vi "Write Start Meas.vi"(8 "error in (no error)":errorcluster, 10 "Start Meas":bool, 11 "Control-Client in":refnum<class "Control-Client.lvclass">) -> (0 "error out":errorcluster, 3 "Control-Client out":refnum<class "Control-Client.lvclass">)   [LabVIEW 2015, in "Control-Client.lvclass"]
uses:
  Control-Client.lvclass
  Control-Client.lvclass/Control-Client.ctl
  dependecies/ControlsVIs/Clusters-def/SERVER-Commands.ctl
  dependecies/ControlsVIs/Clusters-def/Message types.ctl
  dependecies/ControlsVIs/Clusters-def/Def_Vis_Update.ctl
  Experiments/Experiment.lvclass/Experiment.ctl
  Experiments/Experiment.lvclass
  Control-Server/Control-Server.lvclass
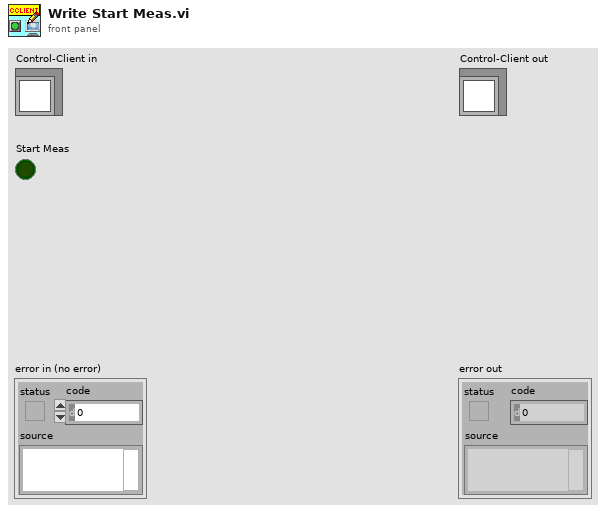
[diagram p1: front panel]
types:
  T1 = typedef "Control-Client.lvclass/Def_Vis_Update.ctl" = cluster{"Data":sgl[][], "timedelays":dbl[], "wavelength":dbl[]}
  T2 = typedef "Message types.ctl" = string
  T3 = typedef "Control-Server.lvclass/SERVER-Commands.ctl" = string
  T4 = cluster{"min I, mm":dbl, "max I, mm":dbl, "Real Optical 0, ps":dbl, "min II, mm":dbl, "max II, mm ":dbl}
  T5 = enum16{"Left Button", "Center Button", "Right Button", "Window Close"}
  T6 = typedef "Control-Client.lvclass/Delays-refs_CLIENT.ctl" = cluster{"# points":refnum<vi>, "Step, ps":refnum<vi>, "OZ, ps":refnum<vi>, "# current":refnum<vi>, "RDT, ps":refnum<vi>, "Total length, ps":refnum<vi>, "Kinetics length, ps":refnum<vi>, "Real zero, ps":refnum<vi>, "# par point":refnum<vi>}
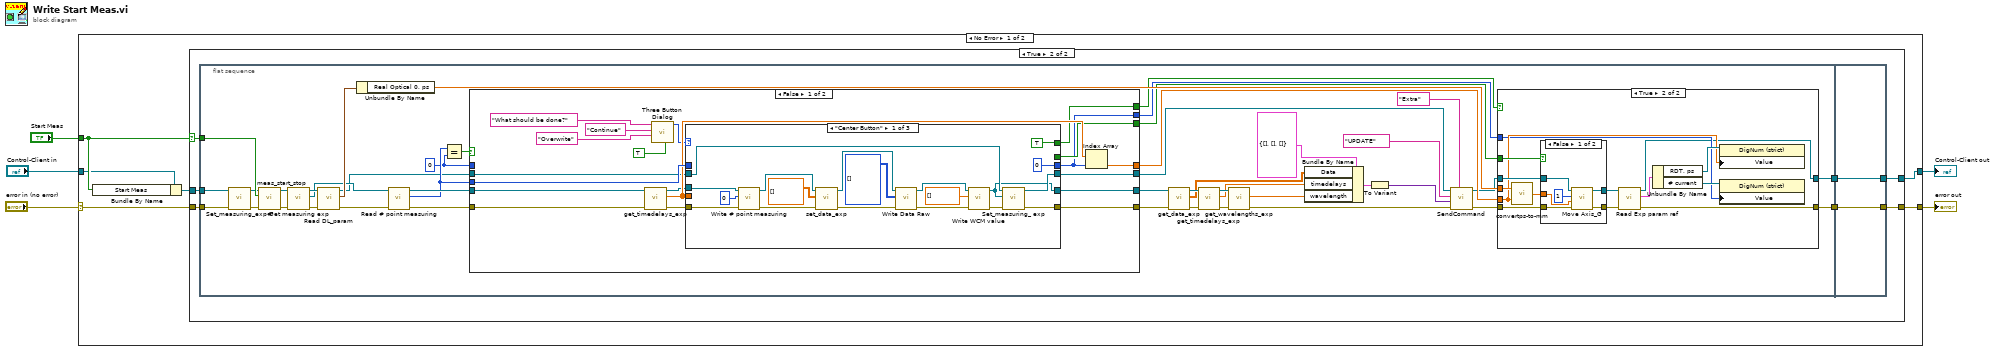
[diagram p0: block diagram]
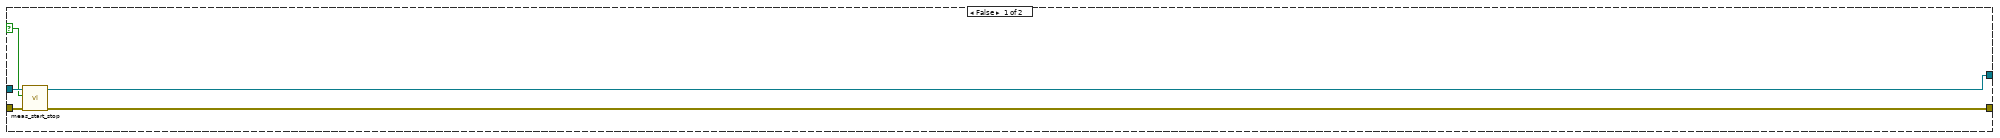
[diagram p2: hidden frame]
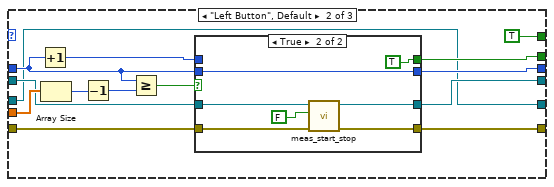
[diagram p5: hidden frame]
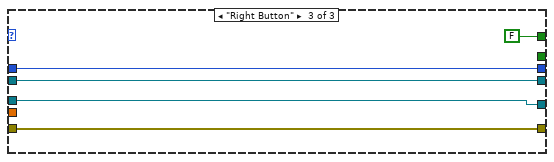
[diagram p7: hidden frame]
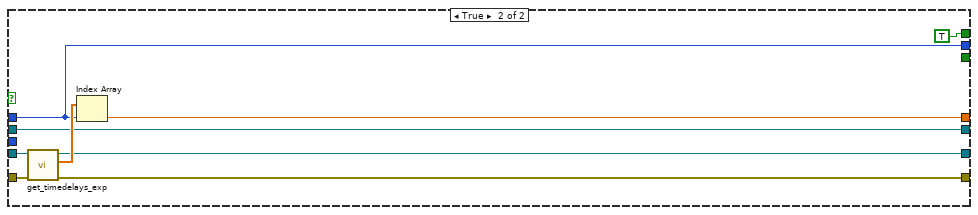
[diagram p8: hidden frame]
diagram:
  n1 = case shown="No Error" "error in (no error)" {
    selector: "error in (no error)" -> [w9 w169]
    tunnel: [w8 w169] -> w4
    tunnel: [w7 w170] -> w2
    tunnel: "Control-Client in" -> [w10 w170]
    tunnel: "Start Meas" -> [w11 _]
    frame No Error {
      n2 = Bundle By Name(cluster=w10, "Start Meas"=w11) -> (w6:refnum<class "Control-Client.lvclass">)
      n3 = case shown="True" w11 {
        selector: w11 -> [w12 w21]
        tunnel: w6 -> [w16 w22]
        tunnel: w9 -> [w15 w23]
        tunnel: [w14 w19] -> w8
        tunnel: [w13 w20] -> w7
        frame False {
          n4 = call "meas_start_stop.vi"("error in (no error)"=w15, "ON/OFF"=w12, "Control-Client in"=w16) -> ("error out"=w14:errorcluster, "Control-Client out"=w13:refnum<class "Control-Client.lvclass">)  [unwired: 7 in]
        }
        frame True {
          n5 = flat-sequence {
            tunnel: [w50] -> w18
            tunnel: [w54] -> w17
            tunnel: w23 -> [w45]
            tunnel: w22 -> [w44]
            tunnel: w21 -> [w56]
            tunnel: [w168] -> w20
            tunnel: w18 -> [w168]
            tunnel: [w167] -> w19
            tunnel: w17 -> [w167]
            frame #0 {
              w52 = 0 ("y")
              n6 = call "Set_measuring_exp#.vi"("error in (no error)"=w45, "Control-Client in"=w44) -> ("error out"=w42:errorcluster, "Control-Client out"=w43:refnum<class "Control-Client.lvclass">)  [unwired: 8 in]
              n7 = call "meas_start_stop.vi"("error in (no error)"=w42, "ON/OFF"=w56, "Control-Client in"=w43) -> ("error out"=w57:errorcluster, "Control-Client out"=w55:refnum<class "Control-Client.lvclass">)  [unwired: 7 in]
              n8 = call "Get measuring exp.vi"("error in (no error)"=w57, "Control-Client in"=w55) -> ("error out"=w47:errorcluster, "Measured experiment"=w61:refnum<class "Experiment.lvclass">, "Control-Client out"=w66:refnum<class "Control-Client.lvclass">)  [unwired: 7 in]
              n9 = call "Read DL_param.vi"("error in (no error)"=w47, "Control-Client in"=w66) -> ("error out"=w46:errorcluster, "DL_param"=w65:T4, "Control-Client out"=w48:refnum<class "Control-Client.lvclass">)  [unwired: 7 in]
              n10 = Unbundle By Name(w65) -> ("Real Optical 0, ps"=w64:dbl)
              n11 = call "Read # point measuring.vi"("error in (no error)"=w46, "Experiment in"=w61) -> ("error out"=w62:errorcluster, "# point measuring"=w59:i32, "Experiment out"=w63:refnum<class "Experiment.lvclass">)  [unwired: 7 in]
              n12 = Equal?(x=w59, y=w52) -> (x = y?=w60:bool)
              n13 = case shown="False" w60 {
                tunnel: w48 -> [w102 w161]
                tunnel: w62 -> [w105 w166]
                tunnel: w63 -> [w108 w165]
                tunnel: [w103 w164] -> w35
                tunnel: [w106 w162] -> w53
                tunnel: w59 -> [w109 _]
                tunnel: [w101 w161] -> w39
                tunnel: [w100 _] -> w58
                tunnel: w52 -> [_ w160]
                tunnel: [w99 w160] -> w51
                tunnel: [w92 TRUE] -> w49
                tunnel: [w91 w158] -> w34
                frame False {
                  n14 = call "get_timedelays_exp.vi"("error in (no error)"=w105, "Experiment.lvclass in"=w108) -> ("error out"=w104:errorcluster, "timedelays"=w107:dbl[], "Experiment.lvclass out"=w98:refnum<class "Experiment.lvclass">)  [unwired: 7 in]
                  n15 = call <vilib>:"Three Button Dialog.vi"("Allow user to close window? (TRUE)"=TRUE, "Center Button Text (\"No\")"="Overwrite" ("F button name (\"Cancel\")"), "Left Button Text (\"Yes\")"="Continue" ("T button name (\"OK\")"), "message"="What should be done?") -> ("Which Button?"=w93:T5)  [unwired: 7 in]
                  n16 = case shown="\"Center Button\"" w93 {
                    tunnel: w98 -> [w127 w129 w153]
                    tunnel: w109 -> [_ w132 w156]
                    tunnel: w107 -> [_ w140 _]
                    tunnel: [0 w139 w156] -> w99
                    tunnel: w104 -> [w125 w135 w155]
                    tunnel: [w123 w134 w155] -> w103
                    tunnel: w102 -> [w120 w136 w157]
                    tunnel: [w124 w133 w157] -> w101
                    tunnel: [_ w137 _] -> w100
                    tunnel: [TRUE TRUE FALSE] -> w92
                    tunnel: [w110 w129 w153] -> w91
                    frame "Center Button" {
                      n17 = call "Write # point measuring.vi"("error in (no error)"=w125, "# point measuring"=0, "Experiment in"=w127) -> ("error out"=w122:errorcluster, "Experiment out"=w121:refnum<class "Experiment.lvclass">)  [unwired: 7 in]
                      n18 = call "set_data_exp.vi"("error in (no error)"=w122, "Data"=dbl[][] [], "Experiment.lvclass in"=w121) -> ("error out"=w118:errorcluster, "Experiment.lvclass out"=w119:refnum<class "Experiment.lvclass">)  [unwired: 7 in]
                      n19 = call-dynamic "Write Data Raw.vi"("error in (no error)"=w118, "Data Raw"=i32[][][][] [], "Experiment in"=w119) -> ("error out"=w117:errorcluster, "Experiment out"=w115:refnum<class "Experiment.lvclass">)  [unwired: 7 in]
                      n20 = call-dynamic "Write WCM value.vi"("error in (no error)"=w117, "WCM value"=sgl[] [], "Experiment in"=w115) -> ("error out"=w116:errorcluster, "Experiment out"=w110:refnum<class "Experiment.lvclass">)  [unwired: 7 in]
                      n21 = call "Set_measuring_ exp.vi"("error in (no error)"=w116, "Experiment"=w110, "Control-Client in"=w120) -> ("error out"=w123:errorcluster, "Control-Client out"=w124:refnum<class "Control-Client.lvclass">)  [unwired: 7 in]
                    }
                    frame "Left Button", Default {
                      n22 = Increment(x=w132) -> (x+1=w141:i32)
                      n23 = Array Size(array=w140) -> (size(s)=w138:i32)
                      n24 = Decrement(x=w138) -> (x-1=w131:i32)
                      n25 = Greater Or Equal?(x=w132, y=w131) -> (x >= y?=w142:bool)
                      n26 = case shown="True" w142 {
                        tunnel: [w145 w152] -> w139
                        tunnel: w141 -> [w145 _]
                        tunnel: w132 -> [_ w152]
                        tunnel: [_ TRUE] -> w137
                        tunnel: w136 -> [w143 w150]
                        tunnel: w135 -> [w144 w148]
                        tunnel: [w144 w147] -> w134
                        tunnel: [w143 w146] -> w133
                        frame False {
                        }
                        frame True {
                          n27 = call "meas_start_stop.vi"("error in (no error)"=w148, "ON/OFF"=FALSE, "Control-Client in"=w150) -> ("error out"=w147:errorcluster, "Control-Client out"=w146:refnum<class "Control-Client.lvclass">)  [unwired: 7 in]
                        }
                      }
                    }
                    frame "Right Button" {
                    }
                  }
                  n28 = Index Array(array=w107, index=w99) -> (element=w106:dbl)
                }
                frame True {
                  n29 = call "get_timedelays_exp.vi"("error in (no error)"=w166, "Experiment.lvclass in"=w165) -> ("error out"=w164:errorcluster, "timedelays"=w163:dbl[], "Experiment.lvclass out"=w158:refnum<class "Experiment.lvclass">)  [unwired: 7 in]
                  n30 = Index Array(array=w163, index=w160) -> (element=w162:dbl)
                }
              }
              n31 = call "get_data_exp.vi"("error in (no error)"=w35, "Experiment.lvclass in"=w34) -> ("error out"=w33:errorcluster, "Data"=w27:sgl[][], "Experiment.lvclass out"=w30:refnum<class "Experiment.lvclass">)  [unwired: 7 in]
              n32 = call "get_timedelays_exp.vi"("error in (no error)"=w33, "Experiment.lvclass in"=w30) -> ("error out"=w32:errorcluster, "timedelays"=w26:dbl[], "Experiment.lvclass out"=w31:refnum<class "Experiment.lvclass">)  [unwired: 7 in]
              n33 = call "get_wavelengths_exp.vi"("error in (no error)"=w32, "Experiment.lvclass in"=w31) -> ("error out"=w24:errorcluster, "wavelengths"=w25:dbl[])  [unwired: 7 in, 1 out]
              n34 = Bundle By Name(cluster=T1 {"Data"=[], "timedelays"=[], "wavelength"=[]}, "Data"=w27, "timedelays"=w26, "wavelength"=w25) -> (w28:T1)
              n35 = To Variant(anything=w28) -> (Variant=w36:variant)
              n36 = call "SendCommand.vi"("Message type"=T2 "Extra", "error in (no error)"=w24, "data"=w36, "Command"=T3 "UPDATE", "Control-Client in"=w39) -> ("error out"=w41:errorcluster, "Control-Client out"=w40:refnum<class "Control-Client.lvclass">)  [unwired: 5 in]
              n37 = case shown="True" w49 {
                tunnel: w64 -> [_ w81]
                tunnel: w40 -> [w68 w80]
                tunnel: w58 -> [_ w79]
                tunnel: w41 -> [w67 w70]
                tunnel: [w67 w69] -> w54
                tunnel: w53 -> [_ w77]
                tunnel: w51 -> [_ w75]
                tunnel: [w68 w74] -> w50
                frame False {
                }
                frame True {
                  n38 = call "convertps-to-mm.vi"("ps"=w77, "Real zero"=w81) -> ("mm"=w82:dbl)
                  n39 = case shown="False" w79 {
                    tunnel: [w87 w90] -> w72
                    tunnel: w82 -> [w86 _]
                    tunnel: [w85 w89] -> w71
                    tunnel: w80 -> [w84 w90]
                    tunnel: w70 -> [w83 w89]
                    frame False {
                      n40 = call "Move Axis_G.vi"("error in (no error)"=w83, "Where, mm"=w86, "Axis"=1, "Control-Client in"=w84) -> ("error out"=w85:errorcluster, "Control-Client out"=w87:refnum<class "Control-Client.lvclass">)  [unwired: 6 in]
                    }
                    frame True {
                    }
                  }
                  n41 = call "Read Exp param ref.vi"("error in (no error)"=w71, "Control-Client in"=w72) -> ("error out"=w69:errorcluster, "Exp param ref"=w73:T6, "Control-Client out"=w74:refnum<class "Control-Client.lvclass">)  [unwired: 7 in]
                  n42 = Unbundle By Name(w73) -> ("RDT, ps"=w78:refnum<vi>, "# current"=w76:refnum<vi>)
                  n43 = property class="DigNum (strict)"(reference=w78, "Value"=w77) -> ()  [unwired: 1 in, 2 out]
                  n44 = property class="DigNum (strict)"(reference=w76, "Value"=w75) -> ()  [unwired: 1 in, 2 out]
                }
              }
            }
            frame #1 {
            }
          }
        }
      }
    }
    frame Error {
    }
  }
  "error out" <- w4
  "Control-Client out" <- w2
